vi "Get Class Name.vi"(1 "GPIB Board in":refnum<class "GPIB Board Design.lvclass">) -> (0 "class name":string)   [LabVIEW 2023, in "GPIB Board Design.lvclass"]
doc: "Get the name of this class."
uses:
  GPIB Board Design.lvclass
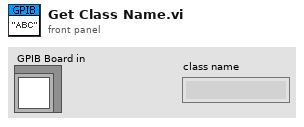
[diagram p1: front panel]
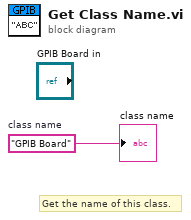
[diagram p0: block diagram]
diagram:
  w1 = "GPIB Board"  # class name
  # "Get the name of this class."
  "class name" <- w1
